vi "exercicio 3.vi"() -> ()   [LabVIEW 2025]
panel:
  in  "Boolean":bool
  in  "F":dbl(slide) scale=0.0..212.0
  out "C":dbl(slide) scale=-100.0..100.0
  out "x*y":dbl
  in  "milliseconds to wait":u32
  out "Numeric":i32
  in  "stop":bool
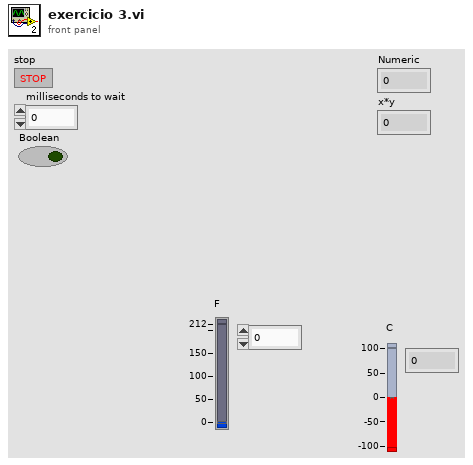
[diagram p1: front panel]
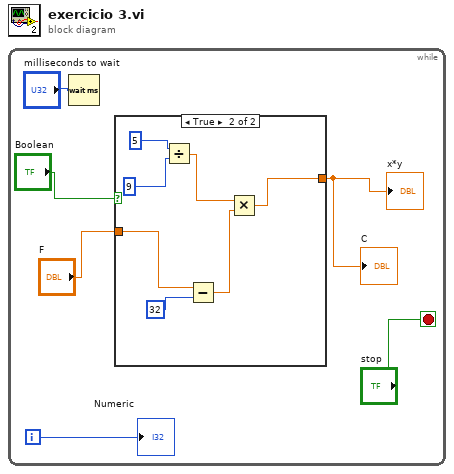
[diagram p0: block diagram]
diagram:
  n1 = while {
    i -> [w4]
    stop <- "stop" stop-if-true
    n2 = Wait (ms)(milliseconds to wait="milliseconds to wait") -> ()  [unwired: 1 out]
    n3 = case shown="True" "Boolean" {
      tunnel: [w7 w9] -> w1
      tunnel: "F" -> [w7 w8]
      frame False {
      }
      frame True {
        n4 = Divide(x=5, y=9) -> (x/y=w12:dbl)
        n5 = Subtract(x=w8, y=32) -> (x-y=w10:dbl)
        n6 = Multiply(x=w12, y=w10) -> (x*y=w9:dbl)
      }
    }
    "x*y" <- w1
    "C" <- w1
    "Numeric" <- w4
  }
